vi "invert_and_blank_caseStruct.vi"(9 "zeroOutput":bool, 10 "invert":bool, 11 "input":i16) -> (3 "output":i16)   [LabVIEW 2016]
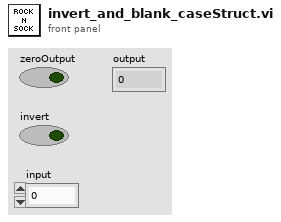
[diagram p1: front panel]
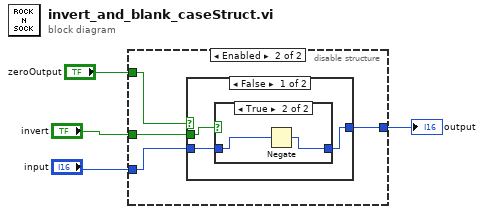
[diagram p0: block diagram]
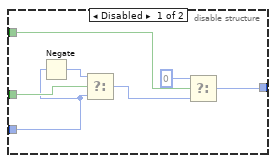
[diagram p2: hidden frame]
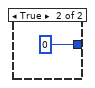
[diagram p4: hidden frame]
diagram:
  n1 = disable-structure shown="Enabled" {
    disable-tunnel: [w11 w14] -> w4
    disable-tunnel: "invert" -> [w8 w13]
    disable-tunnel: "input" -> [w7 w12]
    disable-tunnel: "zeroOutput" -> [w6 w15]
    frame Disabled {
      n2 = Negate(x=w7) -> (-x=w9:i16)
      n3 = Select(t=w9, s=w8, f=w7) -> (s? t:f=w10:i16)
      n4 = Select(t=i16 0, s=w6, f=w10) -> (s? t:f=w11:i16)
    }
    frame Enabled {
      n5 = case shown="False" w15 {
        tunnel: [w17 i16 0] -> w14
        tunnel: w13 -> [w18 _]
        tunnel: w12 -> [w16 _]
        frame False {
          n6 = case shown="True" w18 {
            tunnel: [w19 w20] -> w17
            tunnel: w16 -> [w19 w21]
            frame False {
            }
            frame True {
              n7 = Negate(x=w21) -> (-x=w20:i16)
            }
          }
        }
        frame True {
        }
      }
    }
  }
  "output" <- w4
